vi "Actor Core.vi"(8 "error in":errorcluster, 11 "Calculator Actor in":refnum<class "Calculator Actor.lvclass">) -> (0 "error out":errorcluster, 3 "Actor out":refnum<class "Actor.lvclass">)   [LabVIEW 2015, in "Calculator Actor.lvclass"]
doc: "(<B>Filename</B>: Actor Framework.lvlib:Actor.lvclass:Actor Core.vi)\n\nReceives messages to the actor, reacts to them, and initiates any error handling that may shut the actor down.\n\nDescendant classes may override this VI to append parallel tasks for the actor to complete while it handles messages. Overrides use the Call Parent Method node."
uses:
  Calculator Actor.lvclass
  <vilib>/ActorFramework/Actor/Actor.lvclass
  Addition Actor/Addition Actor Class/Addition Actor.lvclass
  Multiplication Actor/Multiplication Actor Class/Multiplication Actor.lvclass
  Calculator Actor.lvclass/Calculator Actor.ctl
  <vilib>/ActorFramework/Actor/Actor.lvclass/Actor.ctl
  <vilib>/ActorFramework/Message Enqueuer/Message Enqueuer.lvclass/Message Enqueuer.ctl
  <vilib>/ActorFramework/Message Enqueuer/Init from Existing Queue.vi
  <vilib>/ActorFramework/Message Enqueuer/Enqueue.vi
  <vilib>/ActorFramework/Message Priority Queue/Priority Enqueue.vi
  <vilib>/ActorFramework/Message Enqueuer/Message Enqueuer.lvclass
  <vilib>/ActorFramework/Stop Msg/Stop Msg.lvclass
panel:
  out "Result - Multiplication":dbl
  out "Result - Addition":dbl
  in  "Number 2":dbl
  in  "Number 1":dbl
  in  "Calculate":bool
  in  "stop":bool
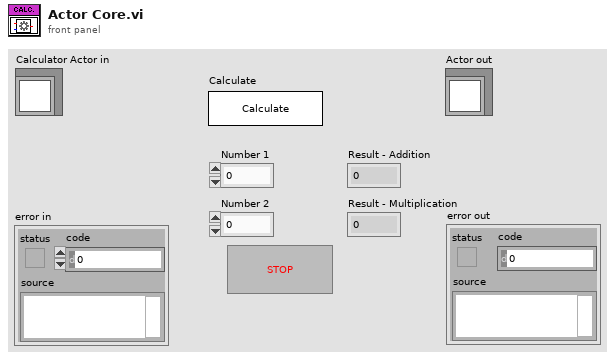
[diagram p1: front panel]
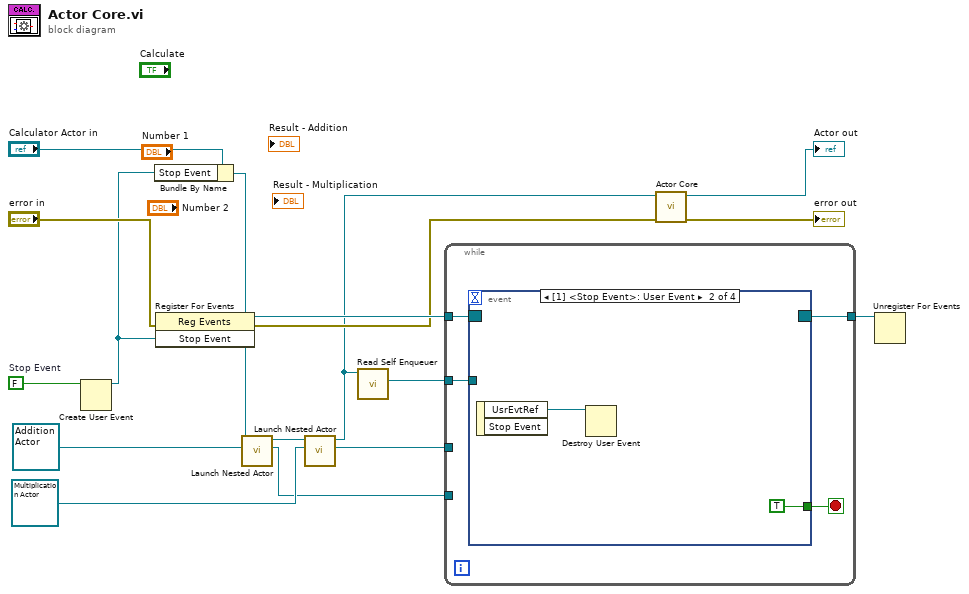
[diagram p0: block diagram]
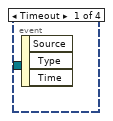
[diagram p2: hidden frame]
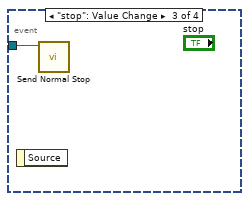
[diagram p3: hidden frame]
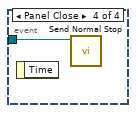
[diagram p4: hidden frame]
diagram:
  w15 = FALSE  # Stop Event
  n1 = Create User Event(user event datatype=w15) -> (user event=w10:refnum<user-event>)  [unwired: 1 in, 1 out]
  n2 = Bundle By Name(cluster="Calculator Actor in", "Stop Event"=w10) -> (w8:refnum<class "Calculator Actor.lvclass">)
  n3 = register-events(error in="error in", w10) -> (reference out=w14:refnum<event-registration>, error out=w12:errorcluster)  [unwired: 1 in]
  n4 = call <vilib>:"Launch Nested Actor.vi"("Nested Actor"=refnum<class "Addition Actor.lvclass"> refnum ("Addition Actor.lvclass"), "Caller Actor in"=w8) -> ("Nested Actor's Enqueuer"=w3:refnum<class "Message Enqueuer.lvclass">, "Caller Actor out"=w6:refnum<class "Calculator Actor.lvclass">)  [unwired: 7 in, 1 out]
  n5 = call <vilib>:"Launch Nested Actor.vi"("Nested Actor"=refnum<class "Multiplication Actor.lvclass"> refnum ("Multiplication Actor.lvclass"), "Caller Actor in"=w6) -> ("Nested Actor's Enqueuer"=w2:refnum<class "Message Enqueuer.lvclass">, "Caller Actor out"=w4:refnum<class "Calculator Actor.lvclass">)  [unwired: 7 in, 1 out]
  n6 = call <vilib>:"Read Self Enqueuer.vi"("Actor"=w4) -> ("Self Enqueuer"=w9:refnum<class "Message Enqueuer.lvclass">)  [unwired: 10 in]
  n7 = while {
    tunnel: w14 -> [w21]
    tunnel: w9 -> [w19]
    tunnel: w3 -> [_]
    tunnel: w2 -> [_]
    tunnel: [w18] -> w1
    stop <- w20 stop-if-true
    n8 = event shown="[1] <Stop Event>: User Event" {
      selector: w21 -> [_ _ _ _]
      dyn-events: [_ _ _ _] -> w18
      timeout: _ -> [_ _ _ _]
      tunnel: [_ TRUE _ _] -> w20
      tunnel: w19 -> [_ _ w24 w25]
      event Timeout {
        n9 = event-data() -> ()  [unwired: 1 in, 3 out]
      }
      event User Event {
        n10 = event-data() -> ("UsrEvtRef"=w22:refnum<user-event>)  [unwired: 1 in, 1 out]
        n11 = Destroy User Event(user event=w22) -> ()  [unwired: 1 in, 1 out]
      }
      event "stop": Value Change {
        n12 = event-data() -> ()  [unwired: 1 in, 1 out]
        n13 = call <vilib>:"Send Normal Stop.vi"("Message Enqueuer"=w24) -> ()  [unwired: 10 in, 1 out]
      }
      event Panel Close {
        n14 = event-data() -> ()  [unwired: 1 in, 1 out]
        n15 = call <vilib>:"Send Normal Stop.vi"("Message Enqueuer"=w25) -> ()  [unwired: 10 in, 1 out]
      }
    }
  }
  n16 = call-parent "Actor Core.vi"("error in"=w12, "Actor in"=w4) -> ("error out"=→"error out":errorcluster, "Actor out"=→"Actor out":refnum<class "Actor.lvclass">)  [unwired: 8 in]
  n17 = Unregister For Events(event registration refnum=w1) -> ()  [unwired: 1 in, 1 out]
